vi "checkError.vi"(8 "error in (no error)":errorcluster, 11 "Monochromator in":refnum<class "Monochromator.lvclass">) -> (0 "error out":errorcluster, 3 "Monochromator out":refnum<class "Monochromator.lvclass">)   [LabVIEW 2016, in "Monochromator.lvclass"]
uses:
  Monochromator.lvclass
  Typedefs/SWStatus.ctl
  MonoStateFactory/MonoStateFactory.lvclass
  Monochromator.lvclass/Monochromator.ctl
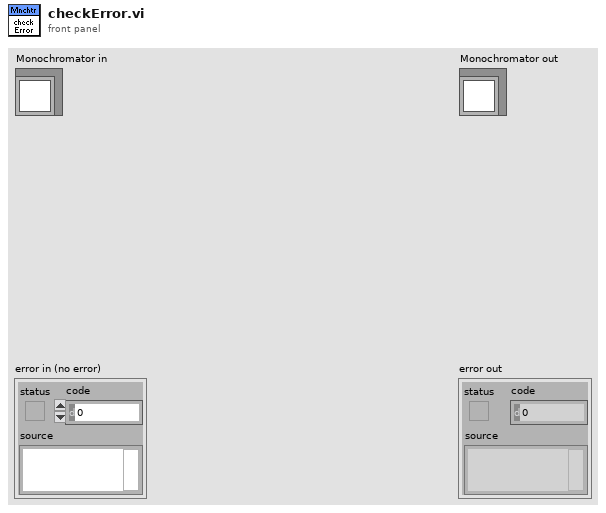
[diagram p1: front panel]
types:
  T1 = typedef "SWStatus.ctl" = enum16{"OfflineState", "ReadyState", "SettingUpState", "FaultState"}
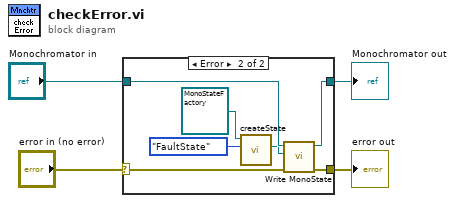
[diagram p0: block diagram]
diagram:
  n1 = case shown="Error" "error in (no error)" {
    selector: "error in (no error)" -> [w5 w11]
    tunnel: [w5 w10] -> w3
    tunnel: [w6 w12] -> w1
    tunnel: "Monochromator in" -> [w6 w13]
    frame No Error {
    }
    frame Error {
      n2 = call "createState.vi"("SWStatus"=SWStatus."FaultState", "MonoStateFactory in"=refnum<class "MonoStateFactory.lvclass"> refnum ("MonoStateFactory.lvclass")) -> ("MonoState.lvclass"=w9:refnum<class "MonoState.lvclass">)  [unwired: 7 in, 2 out]
      n3 = call "Write MonoState.vi"("error in (no error)"=w11, "MonoState.lvclass"=w9, "Monochromator in"=w13) -> ("error out"=w10:errorcluster, "Monochromator out"=w12:refnum<class "Monochromator.lvclass">)  [unwired: 7 in]
    }
  }
  "error out" <- w3
  "Monochromator out" <- w1
